vi "ITestSettings Raw Configuration to Specific Data Type.vi"(8 "error in (no error)":errorcluster, 10 "Raw Config Data":refnum<class "String Database.lvclass">[](array[class]), 11 "IMD Test Settings in":refnum<class "IMD Test Settings.lvclass">) -> (0 "error out":errorcluster, 3 "IMD Test Settings out":refnum<class "IMD Test Settings.lvclass">)   [LabVIEW 2016, in "IMD Test Settings.lvlib" / "IMD Test Settings.lvclass"]
uses:
  IMD Test Settings.lvclass
  C:/Projects/STS/Common/Sequence Automation/Plugins/Test Settings/ITestSettings.lvlibp/ITestSettings.lvclass
  Plugins/String Database.lvlibp/String Database.lvclass
  Controls/IMD Settings Cluster.ctl
  Plugins/Test Settings/ITestSettings.lvlibp/Protected Methods/Read Configuration Dictionary.vi
  Plugins/Test Settings/ITestSettings.lvlibp/Protected Methods/Write Configuration Dictionary.vi
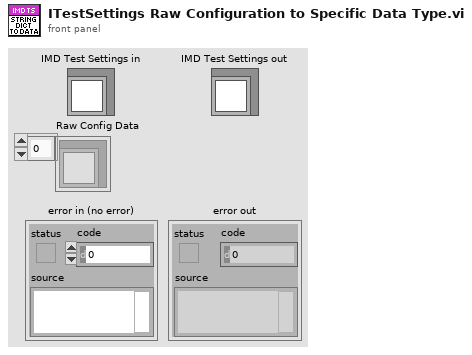
[diagram p1: front panel]
types:
  T1 = typedef "IMD Test Settings.lvlib/IMD Test Settings.lvclass/IMD Settings Cluster.ctl" = cluster{"SG Frequency Offset":dbl, "SA Frequency Offset":dbl, "SA Reference Level":dbl, "2SG Frequency":dbl, "2SG Relative Power Level":dbl, "2SG Waveform Name":string}
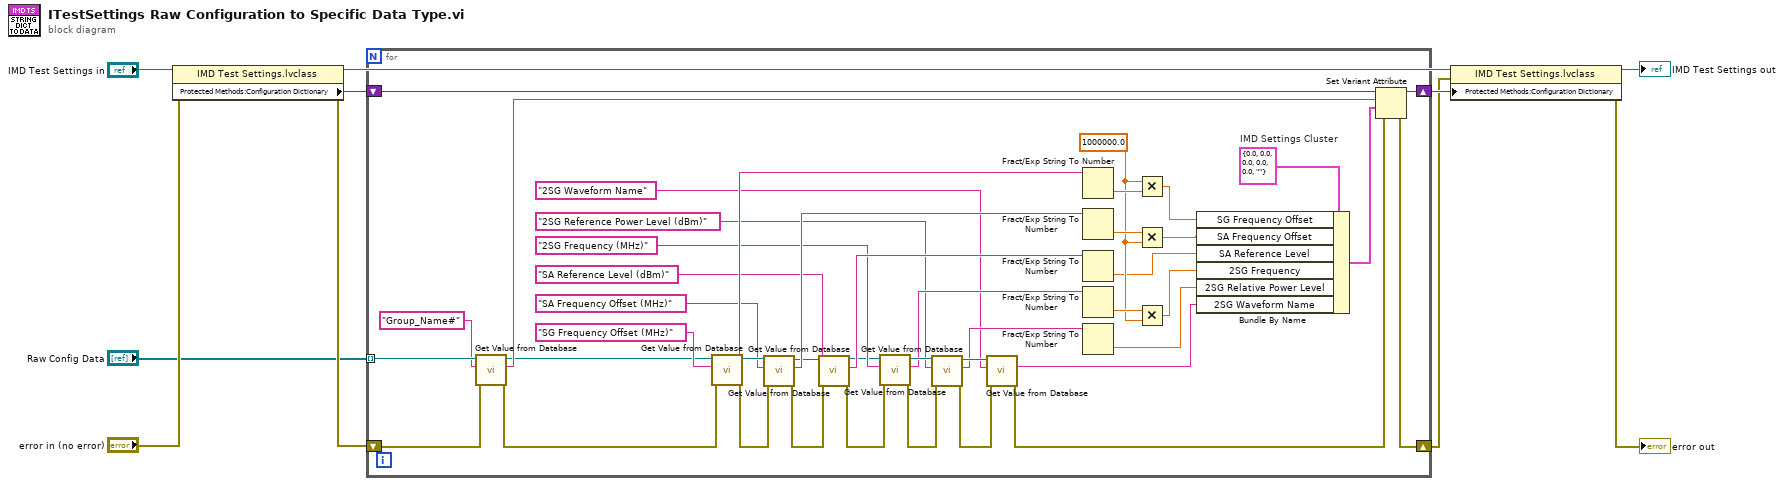
[diagram p0: block diagram]
diagram:
  n1 = property class="IMD Test Settings.lvclass"(reference="IMD Test Settings in", error in="error in (no error)") -> (reference out=w4:refnum<class "IMD Test Settings.lvclass">, error out=w7:errorcluster, "Protected Methods:Configuration Dictionary"=w9:variant)
  n2 = for {
    shift-right: [w52] -> w3
    shift-left: w7 -> [w49]
    shift-right: [w51] -> w5
    shift-left: w9 -> [w53]
    tunnel: "Raw Config Data" -> [w50] mode=indexing
    w24 = 1000000.0 ("x")
    w45 = T1 {"SG Frequency Offset"=0.0, "SA Frequency Offset"=0.0, "SA Reference Level"=0.0, "2SG Frequency"=0.0, "2SG Relative Power Level"=0.0, "2SG Waveform Name"=""}  # IMD Settings Cluster
    n3 = call "Get Value from Database.vi"("error in (no error)"=w49, "Entry Name"="Group_Name#", "Message in"=w50) -> ("error out"=w11:errorcluster, "Entry Value"=w47:string, "Message out"=w19:refnum<class "String Database.lvclass">)  [unwired: 5 in, 1 out]
    n4 = call "Get Value from Database.vi"("error in (no error)"=w11, "Entry Name"="SG Frequency Offset (MHz)", "Message in"=w19) -> ("error out"=w43:errorcluster, "Entry Value"=w41:string, "Message out"=w44:refnum<class "String Database.lvclass">)  [unwired: 5 in, 1 out]
    n5 = call "Get Value from Database.vi"("error in (no error)"=w43, "Entry Name"="SA Frequency Offset (MHz)", "Message in"=w44) -> ("error out"=w35:errorcluster, "Entry Value"=w37:string, "Message out"=w36:refnum<class "String Database.lvclass">)  [unwired: 5 in, 1 out]
    n6 = call "Get Value from Database.vi"("error in (no error)"=w35, "Entry Name"="SA Reference Level (dBm)", "Message in"=w36) -> ("error out"=w28:errorcluster, "Entry Value"=w33:string, "Message out"=w26:refnum<class "String Database.lvclass">)  [unwired: 5 in, 1 out]
    n7 = call "Get Value from Database.vi"("error in (no error)"=w28, "Entry Name"="2SG Frequency (MHz)", "Message in"=w26) -> ("error out"=w30:errorcluster, "Entry Value"=w23:string, "Message out"=w31:refnum<class "String Database.lvclass">)  [unwired: 5 in, 1 out]
    n8 = call "Get Value from Database.vi"("error in (no error)"=w30, "Entry Name"="2SG Reference Power Level (dBm)", "Message in"=w31) -> ("error out"=w29:errorcluster, "Entry Value"=w21:string, "Message out"=w32:refnum<class "String Database.lvclass">)  [unwired: 5 in, 1 out]
    n9 = call "Get Value from Database.vi"("error in (no error)"=w29, "Entry Name"="2SG Waveform Name", "Message in"=w32) -> ("error out"=w12:errorcluster, "Entry Value"=w18:string)  [unwired: 5 in, 2 out]
    n10 = Fract/Exp String To Number(string=w41) -> (number=w40:dbl)  [unwired: 3 in, 1 out]
    n11 = Fract/Exp String To Number(string=w37) -> (number=w38:dbl)  [unwired: 3 in, 1 out]
    n12 = Fract/Exp String To Number(string=w33) -> (number=w15:dbl)  [unwired: 3 in, 1 out]
    n13 = Fract/Exp String To Number(string=w23) -> (number=w25:dbl)  [unwired: 3 in, 1 out]
    n14 = Fract/Exp String To Number(string=w21) -> (number=w17:dbl)  [unwired: 3 in, 1 out]
    n15 = Multiply(x=w24, y=w40) -> (x*y=w13:dbl)
    n16 = Multiply(x=w38, y=w24) -> (x*y=w14:dbl)
    n17 = Multiply(x=w25, y=w24) -> (x*y=w16:dbl)
    n18 = Bundle By Name(cluster=w45, "SG Frequency Offset"=w13, "SA Frequency Offset"=w14, "SA Reference Level"=w15, "2SG Frequency"=w16, "2SG Relative Power Level"=w17, "2SG Waveform Name"=w18) -> (w46:T1)
    n19 = Set Variant Attribute(Variant=w53, name=w47, value=w46, error in=w12) -> (Variant out=w51:variant, error out=w52:errorcluster)  [unwired: 1 out]
  }
  n20 = property class="IMD Test Settings.lvclass"(reference=w4, error in=w3, "Protected Methods:Configuration Dictionary"=w5) -> (reference out=→"IMD Test Settings out":refnum<class "IMD Test Settings.lvclass">, error out=→"error out":errorcluster)
